vi "spDevice_setup.vi"(4 "OffsetB":dbl=-141.0, 5 "Offset":dbl=-209.0, 6 "GainB":dbl=1.0, 7 "Gain":dbl=1.0, 8 "error in":errorcluster, 10 "Blink?":bool, 11 "Trigger":enum32{"Software", "Level", "External"}(radio)=enum."External") -> (0 "error out":errorcluster, 1 "Status window":string="Scanning for Device ...\nFound ADQ214 board: 1", 2 "Sampling Frequency":dbl=400.0, 3 "adq_cu_ptr":u32=322175048)   [LabVIEW 2013]
doc: "Set up the SPDevices ADQ214 digitiser with the following parameters\n - Internal samling clock @400MHz\n - AC coupling on both channels\n - 16-bit unpacked sample format\n - No sample skip.\n\nThe users needs to supply\n - Sofware of external trigger\n - Pretrig/post trig samples (and the number of samples)\n - Whether to blink the front light (indicates machine is working)."
panel:
  in  "OffsetB 2":dbl=-141.0
  in  "GainB 2":dbl=1.0
  in  "Offset 2":dbl=-209.0
  in  "Gain 2":dbl=1.0
  in  "Tab Control":T1(tab)=enum."Sample Format"
  in  "External\nSampling frequency":dbl=400.0 min=20.0 max=400.0 step=1.0
  in  "Clock source (MHz)":T2(radio)=enum."Internal with 10MHz external refference"
  in  "Internal sampling\n frequency":i32(ring) items=["400.000000", "266.666667", "200.000000", "160.000000", "133.333333", "114.285714", "100.000000", "88.888889", "80.000000", "72.727273", "66.666667", "61.538462", "57.142857", "53.333333", "50.000000", "47.058824", "44.444444", "42.105263", "40.000000"]
  in  "Channel A \nCoulpling":enum32{"AC", "DC"}(radio)
  in  "Channel B \nCoulpling":enum32{"AC", "DC"}(radio)
  in  "Level":i32=200 min=-8192 max=8191
  in  "Ch A":bool=TRUE
  in  "Ch B":bool
  in  "Edge":enum32{"Falling", "Rising"}(radio)
  in  "Sample Skip Factor":u32(ring) items=["1", "2", "4", "8", "16", "32", "64", "128", "256", "512", "1024", "2048", "4096", "8192", "16384", "32768", "65536", "131072"]
  in  "Data Format":u32(ring)=1 items=["FORMAT_PACKED_14BIT", "FORMAT_UNPACKED_14BIT", "FORMAT_UNPACKED_16BIT", "FORMAT_UNPACKED_32BIT"]
  in  "PreTrig or HoldOff":u16(ring)=1 items=["Pretrig", "TrigHoldOffSample"]
  in  "Hold off samples":u32 max=2147483648
  in  "Pretrig Samples":u32
  # "-141"
  # "-209"
  # "Channel A"
  # "Channel B"
  # "VI Output"
  # "Channel A"
  # "Channel B"
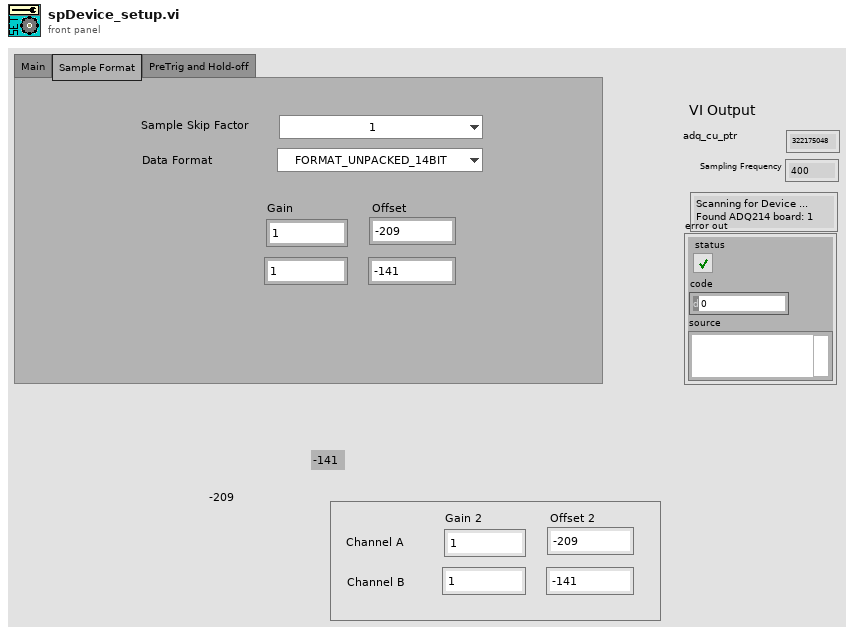
[diagram p1: front panel]
types:
  T1 = enum32{"Main", "Sample Format", "PreTrig and Hold-off"}
  T2 = enum32{"Internal", " External", "Internal with 10MHz external refference"}
  T3 = enum8{"Enabled", "Disabled", "Disabled and Grayed Out"}
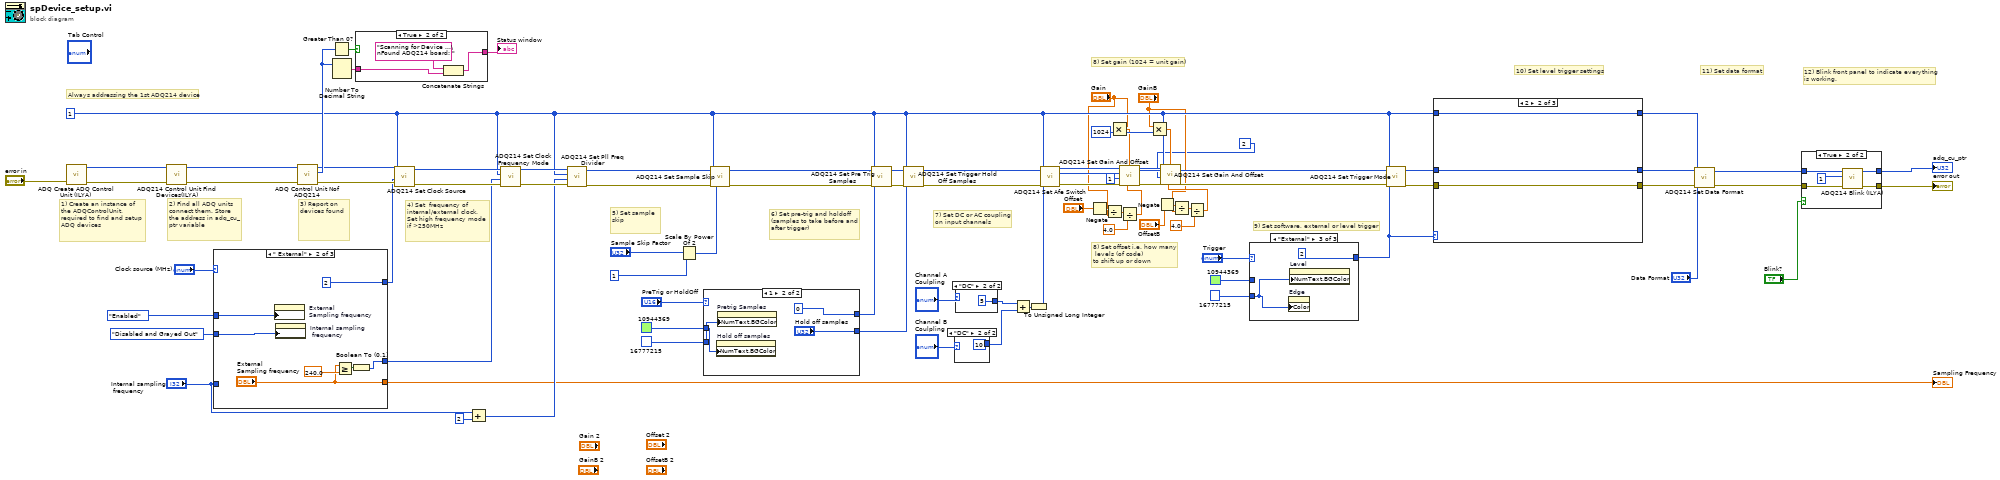
[diagram p0: block diagram]
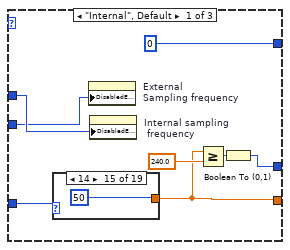
[diagram p3: hidden frame]
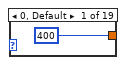
[diagram p4: hidden frame]
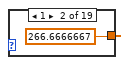
[diagram p5: hidden frame]
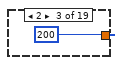
[diagram p6: hidden frame]
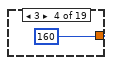
[diagram p7: hidden frame]
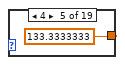
[diagram p8: hidden frame]
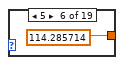
[diagram p9: hidden frame]
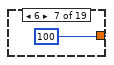
[diagram p10: hidden frame]
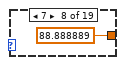
[diagram p11: hidden frame]
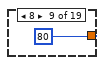
[diagram p12: hidden frame]
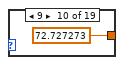
[diagram p13: hidden frame]
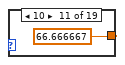
[diagram p14: hidden frame]
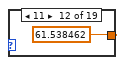
[diagram p15: hidden frame]
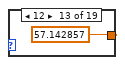
[diagram p16: hidden frame]
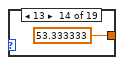
[diagram p17: hidden frame]
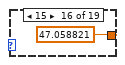
[diagram p18: hidden frame]
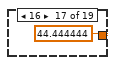
[diagram p19: hidden frame]
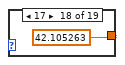
[diagram p20: hidden frame]
diagram:
  w21 = 1
  w79 = 1024
  # "12) Blink front panel to indicate everything\nis working."
  # "6) Set pre-trig and holdoff (samples to take before and after trigger)"
  # "4) Set  frequency of internal/external clock. Set high frequency mode if >250MHz"
  # "5) Set sample skip"
  # "3) Report on devices found"
  # "11) Set data format"
  # "10) Set level trigger settings"
  # "9) Set software, external or level trigger"
  # "8) Set offset i.e. how many\n levels (of code)\nto shift up or down"
  # "8) Set gain (1024 = unit gain)"
  # "7) Set DC or AC coupling\non input channels"
  # "Always addressing the 1st ADQ214 device"
  # "2) Find all ADQ units connect them. Store the address in adq_cu_ptr variable"
  # "1) Create an instance of the ADQControlUnit, required to find and setup ADQ devices"
  n1 = call "ADQ Create ADQ Control Unit (ILYA).vi"("error in (no error)"="error in") -> ("error out"=w85:errorcluster, "function return"=w84:u32)  [unwired: 9 in]
  n2 = call "ADQ214 Control Unit Find Devices(ILYA).vi"("error in (no error)"=w85, "adq_cu_ptr"=w84) -> ("error out"=w41:errorcluster, "adq_cu_ptr out"=w42:u32)  [unwired: 7 in, 1 out]
  n3 = case shown="\" External\"" "Clock source (MHz)" {
    tunnel: [0 2 1] -> w34
    tunnel: "Internal sampling\n frequency" -> [w92 _ w122]
    tunnel: T3."Enabled" ("f") -> [w91 w118 w124]
    tunnel: T3."Disabled and Grayed Out" ("Disabled") -> [w90 w117 w123]
    tunnel: [w87 "External\nSampling frequency" w121] -> w17
    tunnel: [w86 w113 i16 0] -> w16
    frame "Internal", Default {
      n4 = case shown="14" w92 {
        tunnel: [400 266.6666667 200 160 133.3333333 114.285714 100 88.888889 80 72.727273 66.666667 61.538462 57.142857 53.333333 50 47.058821 44.444444 42.105263 40] -> w87
        frame 0, Default {
        }
        frame 1 {
        }
        frame 2 {
        }
        frame 3 {
        }
        frame 4 {
        }
        frame 5 {
        }
        frame 6 {
        }
        frame 7 {
        }
        frame 8 {
        }
        frame 9 {
        }
        frame 10 {
        }
        frame 11 {
        }
        frame 12 {
        }
        frame 13 {
        }
        frame 14 {
        }
        frame 15 {
        }
        frame 16 {
        }
        frame 17 {
        }
        frame 18 {
        }
      }
      n5 = property on="External\nSampling frequency" class="DigNum (strict)"("DisabledEnum"=w90) -> ()  [unwired: 2 in, 2 out]
      n6 = property on="Internal sampling\n frequency" class="Ring (strict)"("DisabledEnum"=w91) -> ()  [unwired: 2 in, 2 out]
      n7 = Greater Or Equal?(x=w87, y=240.0) -> (x >= y?=w89:bool)
      n8 = Boolean To (0,1)(Boolean=w89) -> (0, 1=w86:i16)
    }
    frame " External" {
      n9 = property on="External\nSampling frequency" class="DigNum (strict)"("DisabledEnum"=w118) -> ()  [unwired: 2 in, 2 out]
      n10 = property on="Internal sampling\n frequency" class="Ring (strict)"("DisabledEnum"=w117) -> ()  [unwired: 2 in, 2 out]
      n11 = Greater Or Equal?(x="External\nSampling frequency", y=240.0) -> (x >= y?=w116:bool)
      n12 = Boolean To (0,1)(Boolean=w116) -> (0, 1=w113:i16)
    }
    frame "Internal with 10MHz external refference" {
      n13 = case shown="3" w122 {
        tunnel: [400 266.6666667 200 160 133.3333333 114.285714 100 88.888889 80 72.727273 66.666667 61.538462 57.142857 53.333333 50 47.058821 44.444444 42.105263 40] -> w121
        frame 0, Default {
        }
        frame 1 {
        }
        frame 2 {
        }
        frame 3 {
        }
        frame 4 {
        }
        frame 5 {
        }
        frame 6 {
        }
        frame 7 {
        }
        frame 8 {
        }
        frame 9 {
        }
        frame 10 {
        }
        frame 11 {
        }
        frame 12 {
        }
        frame 13 {
        }
        frame 14 {
        }
        frame 15 {
        }
        frame 16 {
        }
        frame 17 {
        }
        frame 18 {
        }
      }
      n14 = property on="External\nSampling frequency" class="DigNum (strict)"("DisabledEnum"=w123) -> ()  [unwired: 2 in, 2 out]
      n15 = property on="Internal sampling\n frequency" class="Ring (strict)"("DisabledEnum"=w124) -> ()  [unwired: 2 in, 2 out]
    }
  }
  "Sampling Frequency" <- w17
  n16 = call "ADQ Control Unit Nof ADQ214.vi"("error in (no error)"=w41, "adq_cu_ptr"=w42) -> ("error out"=w39:errorcluster, "function return"=w51:i32, "adq_cu_ptr out"=w40:u32)  [unwired: 7 in]
  n17 = Greater Than 0?(x=w51) -> (x > 0?=w83:bool)
  n18 = Number To Decimal String(number=w51) -> (decimal integer string=w82:string)  [unwired: 1 in]
  n19 = case shown="True" w83 {
    tunnel: ["Scanning for device ...\nDevice not found" w146] -> w43
    tunnel: w82 -> [_ w147]
    frame False {
    }
    frame True {
      n20 = Concatenate Strings("Scanning for Device ...\nFound ADQ214 board: ", w147) -> (w146:string)
    }
  }
  "Status window" <- w43
  n21 = call "ADQ214 Set Clock Source.vi"("error in (no error)"=w39, "source"=w34, "adq214_num"=w21, "adq_cu_ptr"=w40) -> ("error out"=w35:errorcluster, "adq_cu_ptr out"=w36:u32)  [unwired: 5 in, 1 out]
  n22 = Add(x="Internal sampling\n frequency", y=2) -> (x+y=w28:i32)
  n23 = call "ADQ214 Set Clock Frequency Mode.vi"("error in (no error)"=w35, "clockmode"=w16, "adq214_num"=w21, "adq_cu_ptr"=w36) -> ("error out"=w30:errorcluster, "adq_cu_ptr out"=w29:u32)  [unwired: 5 in, 1 out]
  n24 = call "ADQ214 Set Pll Freq Divider.vi"("error in (no error)"=w30, "divider"=w28, "adq214_num"=w21, "adq_cu_ptr"=w29) -> ("error out"=w26:errorcluster, "adq_cu_ptr out"=w27:u32)  [unwired: 5 in, 1 out]
  n25 = Scale By Power Of 2(n="Sample Skip Factor", x=u32 1) -> (x*2^n=w72:u32)
  n26 = case shown="1" "PreTrig or HoldOff" {
    tunnel: ["Pretrig Samples" u32 0 ("Pre trig")] -> w69
    tunnel: [u32 0 ("Trig hold off") "Hold off samples"] -> w50
    tunnel: u32 10944369 -> [w150 w154]
    tunnel: u32 16777215 -> [w149 w153]
    frame 0, Default {
      n27 = property on="Hold off samples" class="DigNum (strict)"("NumText.BGColor"=w149) -> ()  [unwired: 2 in, 2 out]
      n28 = property on="Pretrig Samples" class="DigNum (strict)"("NumText.BGColor"=w150) -> ()  [unwired: 2 in, 2 out]
    }
    frame 1 {
      n29 = property on="Hold off samples" class="DigNum (strict)"("NumText.BGColor"=w154) -> ()  [unwired: 2 in, 2 out]
      n30 = property on="Pretrig Samples" class="DigNum (strict)"("NumText.BGColor"=w153) -> ()  [unwired: 2 in, 2 out]
    }
  }
  n31 = call "ADQ214 Set Sample Skip.vi"("error in (no error)"=w26, "skipfactor"=w72, "adq214_num"=w21, "adq_cu_ptr"=w27) -> ("error out"=w70:errorcluster, "adq_cu_ptr out"=w71:u32)  [unwired: 5 in, 1 out]
  n32 = call "ADQ214 Set Pre Trig Samples.vi"("error in (no error)"=w70, "PreTrigSamples"=w69, "adq214_num"=w21, "adq_cu_ptr"=w71) -> ("error out"=w53:errorcluster, "adq_cu_ptr out"=w52:u32)  [unwired: 5 in, 1 out]
  n33 = call "ADQ214 Set Trigger Hold Off Samples.vi"("error in (no error)"=w53, "TriggerHoldOffSamples"=w50, "adq214_num"=w21, "adq_cu_ptr"=w52) -> ("error out"=w49:errorcluster, "adq_cu_ptr out"=w48:u32)  [unwired: 5 in, 1 out]
  n34 = case shown="\"DC\"" "Channel B \nCoulpling" {
    tunnel: [0 10] -> w80
    frame "AC", Default {
    }
    frame "DC" {
    }
  }
  n35 = case shown="\"DC\"" "Channel A \nCoulpling" {
    tunnel: [0 5] -> w76
    frame "AC", Default {
    }
    frame "DC" {
    }
  }
  n36 = Add(x=w76, y=w80) -> (x+y=w75:i32)
  n37 = To Unsigned Long Integer(number=w75) -> (unsigned 32bit integer=w68:u32)
  n38 = call "ADQ214 Set Afe Switch.vi"("error in (no error)"=w49, "afemask"=w68, "adq214_num"=w21, "adq_cu_ptr"=w48) -> ("error out"=w64:errorcluster, "adq_cu_ptr out"=w63:u32)  [unwired: 5 in, 1 out]
  n39 = Negate(x="Offset") -> (-x=w14:dbl)
  n40 = Divide(x=w14, y="Gain") -> (x/y=w12:dbl)
  n41 = Multiply(x="Gain", y=w79) -> (x*y=w66:dbl)
  n42 = Divide(x=w12, y=4.0) -> (x/y=w10:dbl)
  n43 = call "ADQ214 Set Gain And Offset.vi"("Offset"=w10, "Gain"=w66, "error in (no error)"=w64, "channel"=u8 1, "adq212_num"=w21, "adq_cu_ptr"=w63) -> ("error out"=w65:errorcluster, "adq_cu_ptr out"=w62:u32)  [unwired: 3 in, 1 out]
  n44 = Multiply(x="GainB", y=w79) -> (x*y=w67:dbl)
  n45 = Negate(x="OffsetB") -> (-x=w7:dbl)
  n46 = Divide(x=w7, y="GainB") -> (x/y=w8:dbl)
  n47 = Divide(x=w8, y=4.0) -> (x/y=w5:dbl)
  n48 = call "ADQ214 Set Gain And Offset.vi"("Offset"=w5, "Gain"=w67, "error in (no error)"=w65, "channel"=u8 2, "adq212_num"=w21, "adq_cu_ptr"=w62) -> ("error out"=w38:errorcluster, "adq_cu_ptr out"=w37:u32)  [unwired: 3 in, 1 out]
  n49 = case shown="\"External\"" "Trigger" {
    tunnel: [1 3 2] -> w59
    tunnel: u32 10944369 -> [_ w163 _]
    tunnel: u32 16777215 -> [w161 _ w165]
    frame "Software", Default {
      n50 = property on="Edge" class="RadioBtnsControl (strict)"("Color"=w161) -> ()  [unwired: 2 in, 2 out]
      n51 = property on="Level" class="DigNum (strict)"("NumText.BGColor"=w161) -> ()  [unwired: 2 in, 2 out]
    }
    frame "Level" {
      n52 = property on="Edge" class="RadioBtnsControl (strict)"("Color"=w163) -> ()  [unwired: 2 in, 2 out]
      n53 = property on="Level" class="DigNum (strict)"("NumText.BGColor"=w163) -> ()  [unwired: 2 in, 2 out]
    }
    frame "External" {
      n54 = property on="Edge" class="RadioBtnsControl (strict)"("Color"=w165) -> ()  [unwired: 2 in, 2 out]
      n55 = property on="Level" class="DigNum (strict)"("NumText.BGColor"=w165) -> ()  [unwired: 2 in, 2 out]
    }
  }
  n56 = call "ADQ214 Set Trigger Mode.vi"("error in (no error)"=w38, "trig_mode"=w59, "adq214_num"=w21, "adq_cu_ptr"=w37) -> ("error out"=w58:errorcluster, "adq_cu_ptr out"=w57:u32)  [unwired: 5 in, 1 out]
  n57 = case shown="2" w59 {
    tunnel: w58 -> [w167 w170 w188]
    tunnel: w57 -> [w169 w172 w187]
    tunnel: w21 -> [w168 w171 w177]
    tunnel: [w169 w172 w173] -> w55
    tunnel: [w168 w171 w177] -> w44
    tunnel: [w167 w170 w174] -> w56
    frame 1, Default {
    }
    frame 2 {
    }
    frame 3 {
      n58 = call "ADQ214 Set Lvl Trig Level.vi"("error in (no error)"=w188, "level"="Level", "adq214_num"=w177, "adq_cu_ptr"=w187) -> ("error out"=w185:errorcluster, "adq_cu_ptr out"=w184:u32)  [unwired: 5 in, 1 out]
      n59 = call "ADQ214 Set Lvl Trig Edge.vi"("error in (no error)"=w185, "edge"="Edge", "adq214_num"=w177, "adq_cu_ptr"=w184) -> ("error out"=w175:errorcluster, "adq_cu_ptr out"=w178:u32)  [unwired: 5 in, 1 out]
      n60 = Boolean To (0,1)(Boolean="Ch B") -> (0, 1=w181:i16)
      n61 = Boolean To (0,1)(Boolean="Ch A") -> (0, 1=w179:i16)
      n62 = Add(x=w179, y=w181) -> (x+y=w176:i16)
      n63 = call "ADQ214 Set Lvl Trig Channel.vi"("error in (no error)"=w175, "channel"=w176, "adq214_num"=w177, "adq_cu_ptr"=w178) -> ("error out"=w174:errorcluster, "adq_cu_ptr out"=w173:u32)  [unwired: 5 in, 1 out]
    }
  }
  n64 = call "ADQ214 Set Data Format.vi"("error in (no error)"=w56, "format"="Data Format", "adq214_num"=w44, "adq_cu_ptr"=w55) -> ("error out"=w20:errorcluster, "adq_cu_ptr out"=w19:u32)  [unwired: 5 in, 1 out]
  n65 = case shown="True" "Blink?" {
    tunnel: [w189 w194] -> w47
    tunnel: [w190 w193] -> w18
    tunnel: w19 -> [w190 w192]
    tunnel: w20 -> [w189 w191]
    frame False {
    }
    frame True {
      n66 = call "ADQ214 Blink (ILYA).vi"("error in (no error)"=w191, "adq214_num"=1, "adq_cu_ptr in"=w192) -> ("error out"=w194:errorcluster, "adq_cu_ptr"=w193:u32)  [unwired: 6 in, 1 out]
    }
  }
  "error out" <- w47
  "adq_cu_ptr" <- w18
